vi "get UI reference.vi"(8 "error in":errorcluster, 11 "cosmetic changes in":refnum<class "cosmetic changes.lvclass">) -> (0 "error out":errorcluster, 2 "VI Refnum":refnum<vi>, 3 "cosmetic changes out":refnum<class "cosmetic changes.lvclass">)   [LabVIEW 2013, in "cosmetic changes.lvclass"]
uses:
  cosmetic changes.lvclass
  cosmetic ui.vi
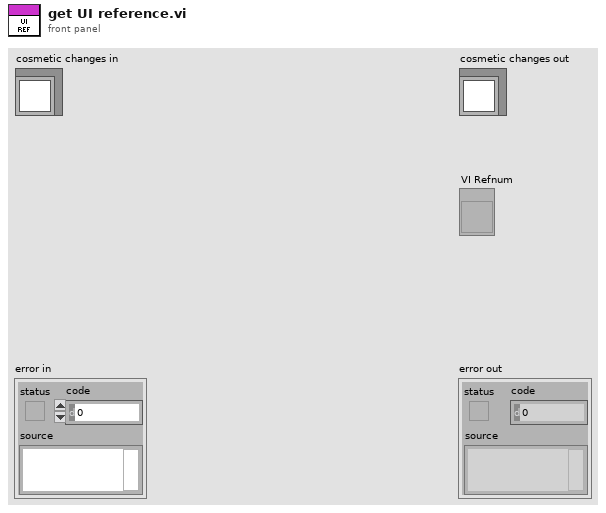
[diagram p1: front panel]
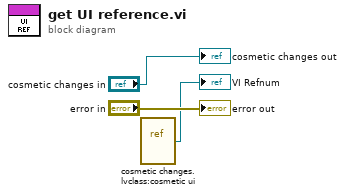
[diagram p0: block diagram]
diagram:
  n1 = vi-ref "cosmetic changes.lvclass:cosmetic ui.vi"() -> (→"VI Refnum":refnum<vi>)
  "error out" <- "error in"
  "cosmetic changes out" <- "cosmetic changes in"
